vi "Get String.vi"(5 "use temporary file? (F)":bool, 7 "data type of variable":string, 8 "error in":errorcluster, 10 "variable name":string, 11 "GOLPI ref. in":T1={"pipe handle"={"lv_proc.dll file path"=path "", "process instance handle"=[], "debug mode"=FALSE, "debug data"=[]}, "fast read timeout [ms]"=500, "fast read settle time [ms]"=10, "fast read to multiple [ms]"=1, "max elements per input line"=100, "slow read timeout [ms]"=5000, "stdin double format specifier"="%_16e", "max elements per stdout output column"=100, "console mode bitstream"=FALSE, "bitstream first read timeout [ms]"=1000, "bitstream read timeout [ms]"=50, "struct transfer possible"=FALSE, "matlab mode"=FALSE, "var pipe write timeout [ms]"=5000, "variable pipe mode"=FALSE, "variable pipe buffer size [Bytes]"=10000000, "variable pipe block size [Bytes]"=1000000} {"variable pipe block size [Bytes]" format="%.0p"; "variable pipe buffer size [Bytes]" format="%.0p"}) -> (0 "error out":errorcluster, 2 "value":string, 3 "GOLPI ref. out":T1={"pipe handle"={"lv_proc.dll file path"=path "", "process instance handle"=[], "debug mode"=FALSE, "debug data"=[]}, "fast read timeout [ms]"=500, "fast read settle time [ms]"=10, "fast read to multiple [ms]"=1, "max elements per input line"=100, "slow read timeout [ms]"=5000, "stdin double format specifier"="%_16e", "max elements per stdout output column"=100, "console mode bitstream"=FALSE, "bitstream first read timeout [ms]"=1000, "bitstream read timeout [ms]"=50, "struct transfer possible"=FALSE, "matlab mode"=FALSE, "var pipe write timeout [ms]"=5000, "variable pipe mode"=FALSE, "variable pipe buffer size [Bytes]"=10000000, "variable pipe block size [Bytes]"=1000000} {"variable pipe block size [Bytes]" format="%.0p"; "variable pipe buffer size [Bytes]" format="%.0p"})   [LabVIEW 2020, in "GOLPI library.lvlib"]
doc: "Part of polymorph Get Variable.vi"
uses:
  GOLPI library.lvlib
  Public/GOLPI reference Type Def.ctl
  LV Process source distribution/Pipe Handle.ctl
  Type Definitions/Bitstream Data Type.ctl
  Type Definitions/Custom Error Codes Enum Type Def.vi
  LV Process source distribution/LV Process library.lvlib
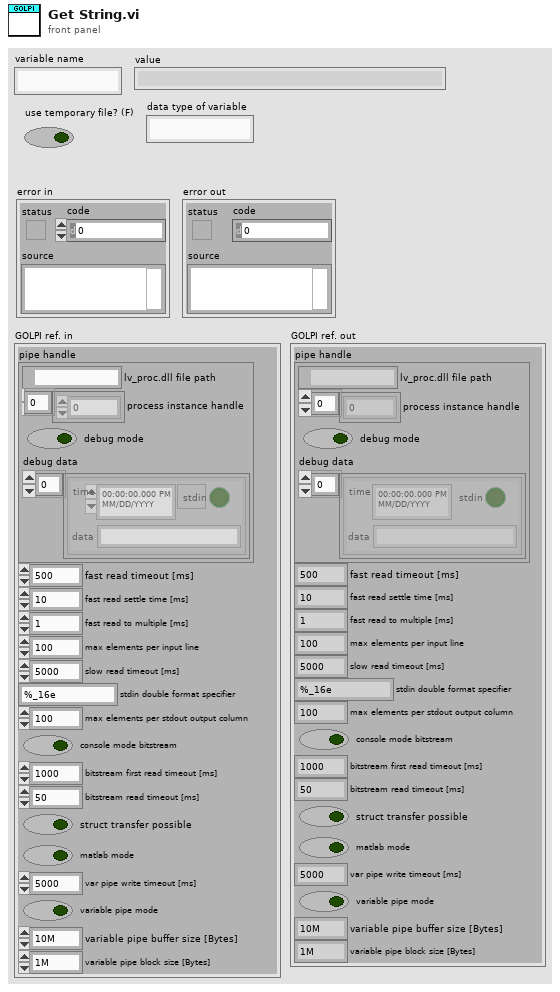
[diagram p1: front panel]
types:
  T1 = typedef "GOLPI library.lvlib/GOLPI reference Type Def.ctl" = cluster{"pipe handle":T2, "fast read timeout [ms]":u32, "fast read settle time [ms]":u32, "fast read to multiple [ms]":u32, "max elements per input line":u32, "slow read timeout [ms]":u32, "stdin double format specifier":string, "max elements per stdout output column":u32, "console mode bitstream":bool, "bitstream first read timeout [ms]":u32, "bitstream read timeout [ms]":u32, "struct transfer possible":bool, "matlab mode":bool, "var pipe write timeout [ms]":u32, "variable pipe mode":bool, "variable pipe buffer size [Bytes]":u32, "variable pipe block size [Bytes]":u32}
  T2 = typedef "LV Process library.lvlib/Pipe Handle.ctl" = cluster{"lv_proc.dll file path":path, "process instance handle":u32[], "debug mode":bool, "debug data":cluster{"time":timestamp, "stdin":bool, "data":string}[]}
  T3 = typedef "GOLPI library.lvlib/Custom Error Codes Enum Type Def.vi" = enum16{"no error", "00 working directory PAR1 missing", "01 octave binary PAR1 missing", "02 octave report error PAR1", "03 empty output last cmd PAR1", "04 missing temporary file PAR1", "05 pwd PAR 1 not exist", "06 oct package not installed", "07 octave default binary missing", "10 var PAR1 not string, vect", "11 var PAR1 not num, scal, ~compl", "12 var PAR1 not num, scal, compl", "13 var PAR1 not num, vect, ~compl", "14 var PAR1 not num, vect, compl", "15 var PAR1 not num, mat, ~compl", "16 var PAR1 not num, mat, ~compl", "30 read timeout", "60 bitstream transport failed", "61 bitstream decode error PAR1", "62 bitstream cannot be set", "70 struct transfer not possible", "80 struct: cluster elem. PAR1 not implem.", "81 struct: structure field PAR1 not implem.", "82 struct: size mismatch of PAR1", "83 struct: type mismatch of PAR1", "98 internal error", "99 not finished", "90 Not supported in Matlab mode", "91 Matlab variable transfer error", "92 Matlab Script Error"}
  T4 = typedef "GOLPI library.lvlib/Bitstream Data Type.ctl" = enum16{"dummy", "int", "uint", "float", "complex", "str", "real numeric"}
  T5 = typedef "GOLPI library.lvlib/Transfer Mode.ctl" = enum16{"Matlab", "stdio", "temp file", "bitstream", "pipe"}
  T6 = typedef "GOLPI library.lvlib/Bitstream Data.ctl" = cluster{"double":dbl[][], "cplx double":cdb[][], "int64":i64[][], "uint64":u64[][], "str":string[], "data type":T4}
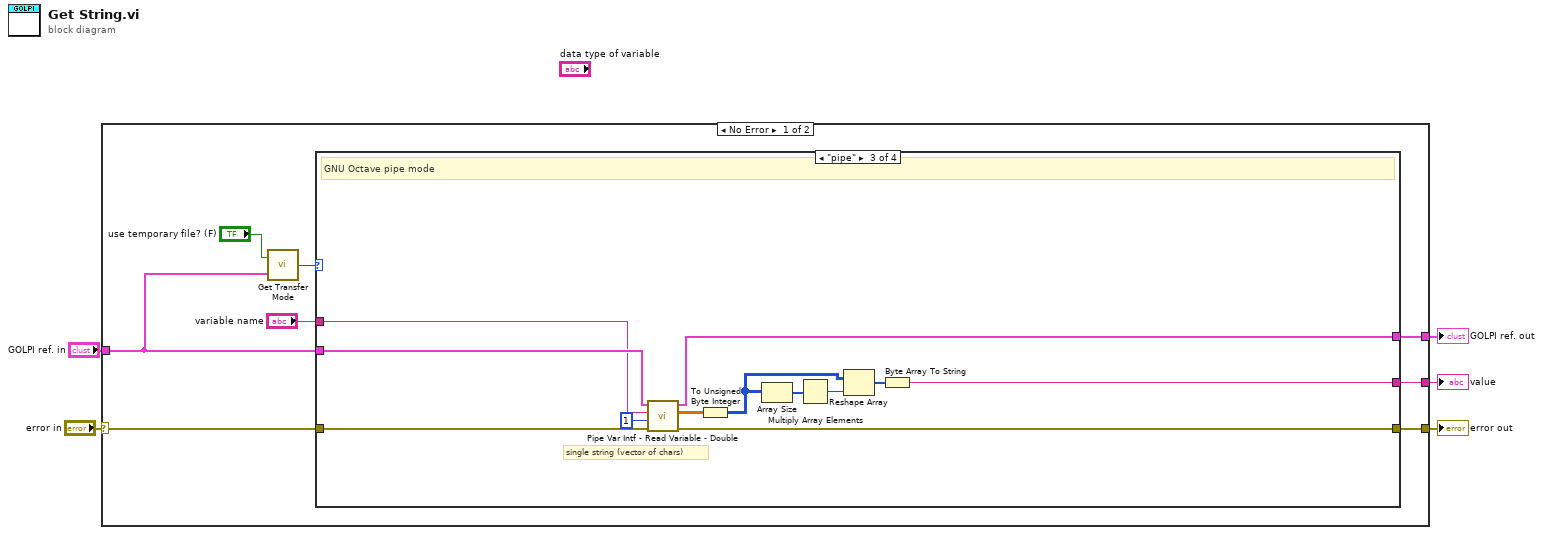
[diagram p0: block diagram]
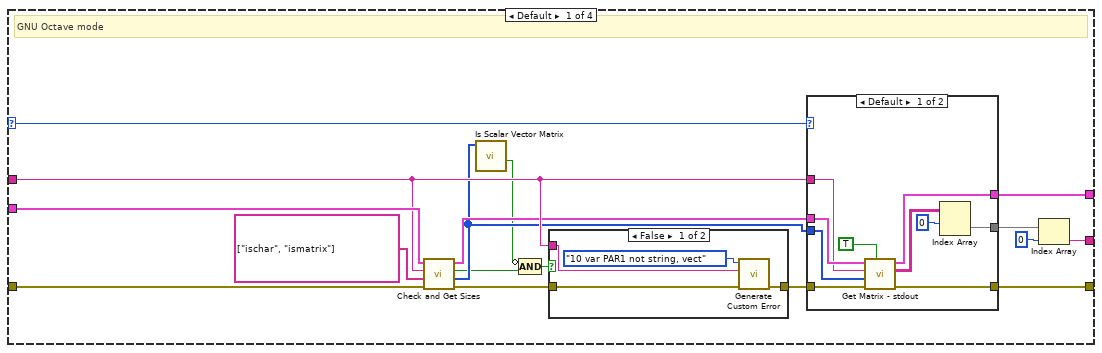
[diagram p2: hidden frame]
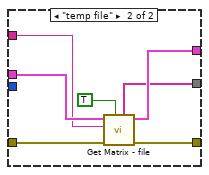
[diagram p3: hidden frame]
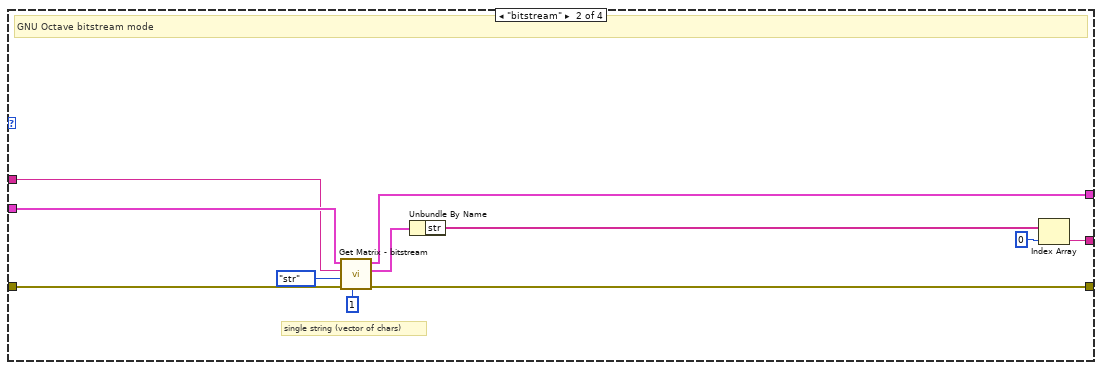
[diagram p5: hidden frame]
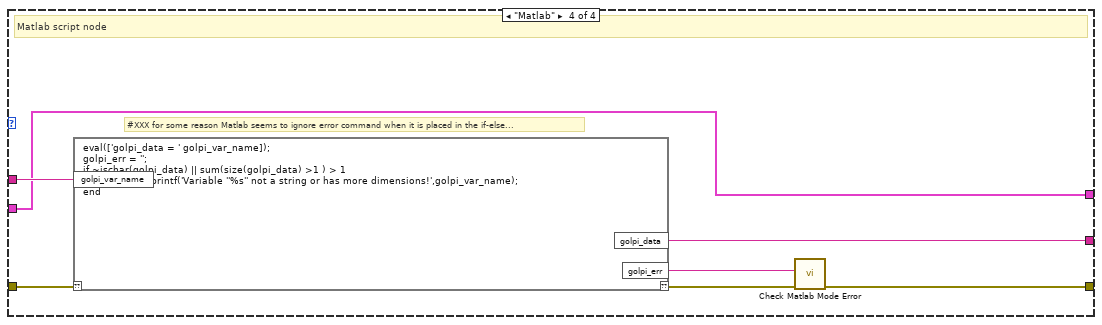
[diagram p6: hidden frame]
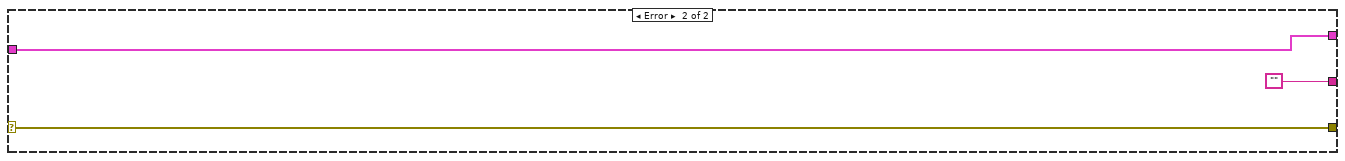
[diagram p7: hidden frame]
diagram:
  n1 = case shown="No Error" "error in" {
    selector: "error in" -> [w13 w84]
    tunnel: [w11 w84] -> w5
    tunnel: [w10 ""] -> w4
    tunnel: "GOLPI ref. in" -> [w8 w83]
    tunnel: [w12 w83] -> w1
    frame No Error {
      n2 = call "Get Transfer Mode.vi"("GOLPI ref."=w8, "use temporary file? (F)"="use temporary file? (F)") -> ("mode"=w7:T5)
      n3 = case shown="\"pipe\"" w7 {
        selector: w7 -> [w14 _ _ _]
        tunnel: w13 -> [w30 w63 w75 w82]
        tunnel: [w29 w62 w74 w80] -> w12
        tunnel: [w26 w59 w73 w77] -> w11
        tunnel: [w25 w58 w64 w76] -> w10
        tunnel: w8 -> [w24 w57 w72 w80]
        tunnel: "variable name" -> [w23 w56 w71 w81]
        frame Default {
          # "GNU Octave mode"
          n4 = call "Check and Get Sizes.vi"("error in (no error)"=w30, "test commands"=string[] ["ischar", "ismatrix"], "variable name"=w23, "GOLPI ref. in"=w24) -> ("error out"=w22:errorcluster, "octave sizes"=w18:i32[], "all tests OK?"=w17:bool, "GOLPI ref. out"=w19:T1)  [unwired: 4 in]
          n5 = call "Is Scalar Vector Matrix.vi"("octave sizes"=w18) -> ("is matrix?"=w15:bool)  [unwired: 5 in, 5 out]
          n6 = Compound Arithmetic op=AND(invert w15, w17) -> (w16:bool)
          n7 = case shown="False" w16 {
            tunnel: [w50 w52] -> w20
            tunnel: w22 -> [w51 w52]
            tunnel: w23 -> [w49 _]
            frame False {
              n8 = call "Generate Custom Error.vi"("error in"=w51, "PAR1"=w49, "GOLPI error"=Custom_Error_Codes_Enum_Type_Def.vi."10 var PAR1 not string, vect" ("Enum")) -> ("error out"=w50:errorcluster)  [unwired: 8 in]
            }
            frame True {
            }
          }
          n9 = case shown="Default" w14 {
            tunnel: w20 -> [w40 w47]
            tunnel: [w39 w45] -> w26
            tunnel: w19 -> [w38 w46]
            tunnel: [w37 w44] -> w29
            tunnel: w23 -> [w35 w42]
            tunnel: w18 -> [w34 _]
            tunnel: [w31 w41] -> w27
            frame Default {
              n10 = call "Get Matrix - stdout.vi"("is string?"=TRUE ("is string"), "error in (no error)"=w40, "octave sizes"=w34, "variable name"=w35, "GOLPI ref. in"=w38) -> ("error out"=w39:errorcluster, "array"=w32:string[][], "GOLPI ref. out"=w37:T1)  [unwired: 4 in]
              n11 = Index Array(array=w32, index (row)=0) -> (element=w31:string[])  [unwired: 1 in]
            }
            frame "temp file" {
              n12 = call "Get Matrix - file.vi"("is string?"=TRUE ("is string"), "error in (no error)"=w47, "variable name"=w42, "GOLPI ref. in"=w46) -> ("error out"=w45:errorcluster, "GOLPI ref. out"=w44:T1, "string array"=w41:string[])  [unwired: 3 in, 2 out]
            }
          }
          n13 = Index Array(array=w27, index=0 ("index (row)")) -> (element=w25:string)
        }
        frame "bitstream" {
          # "single string (vector of chars)"
          # "GNU Octave bitstream mode"
          n14 = call "Get Matrix - bitstream.vi"("max dimensions (0: scalar)"=1, "error in (no error)"=w63, "data type"=Bitstream_Data_Type."str", "variable name"=w56, "GOLPI ref. in"=w57) -> ("error out"=w59:errorcluster, "data"=w53:T6, "GOLPI ref. out"=w62:T1)  [unwired: 4 in]
          n15 = Unbundle By Name(w53) -> ("str"=w60:string[])
          n16 = Index Array(array=w60, index=0 ("index (row)")) -> (element=w58:string)
        }
        frame "pipe" {
          # "single string (vector of chars)"
          # "GNU Octave pipe mode"
          n17 = call "Pipe Var Intf - Read Variable - Double.vi"("error in (no error)"=w75, "max dims (0: scalar)"=1 ("max dimensions (0: scalar)"), "variable name"=w71, "GOLPI ref. in"=w72) -> ("error out"=w73:errorcluster, "data out"=w69:dbl[][], "GOLPI ref. out"=w74:T1)  [unwired: 5 in]
          n18 = To Unsigned Byte Integer(number=w69) -> (unsigned 8bit integer=w66:u8[][])
          n19 = Array Size(array=w66) -> (size(s)=w68:i32[])
          n20 = Multiply Array Elements(1:w68) -> (0:w67:i32)
          n21 = Reshape Array(w66, w67) -> (w65:u8[])
          n22 = Byte Array To String(unsigned byte array=w65) -> (string=w64:string)
        }
        frame "Matlab" {
          # "#XXX for some reason Matlab seems to ignore error command when it is placed in the if-else..."
          # "Matlab script node"
          n23 = script code="eval(['golpi_data = ' golpi_var_name]);\ngolpi_err = '';\nif ~ischar(golpi_data) || sum(size(golpi_data) >1 ) > 1\n  golpi_err = sprintf('Variable ''%s'' not a string or has more dimensions!',golpi_var_name);\nend"("??"=w82, "golpi_var_name"=w81) -> ("??"=w79:errorcluster, "golpi_data"=w76:string, "golpi_err"=w78:string)
          n24 = call "Check Matlab Mode Error.vi"("error in"=w79, "custom error string (empty)"=w78) -> ("error out"=w77:errorcluster)  [unwired: 9 in]
        }
      }
    }
    frame Error {
    }
  }
  "value" <- w4
  "error out" <- w5
  "GOLPI ref. out" <- w1
